vi "proc_append_error.vi"(8 "error in":errorcluster, 11 "code in":i32) -> (0 "error out":errorcluster, 3 "code out":i32)   [LabVIEW 2012]
doc: "Appends LV process error text to error signal."
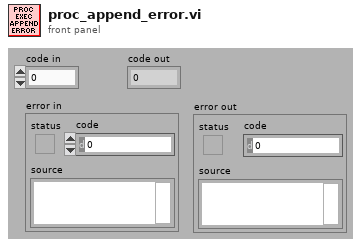
[diagram p1: front panel]
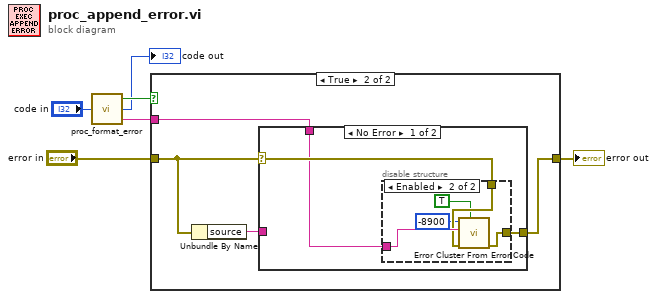
[diagram p0: block diagram]
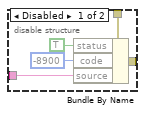
[diagram p3: hidden frame]
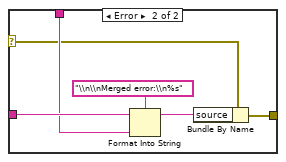
[diagram p4: hidden frame]
diagram:
  n1 = call "proc_format_error.vi"("code in"="code in") -> ("error"=w5:bool, "code out"=→"code out":i32, "error string"=w3:string)
  n2 = case shown="True" w5 {
    tunnel: "error in" -> [w7 w11]
    tunnel: w3 -> [_ w10]
    tunnel: [w7 w8] -> w2
    frame False {
    }
    frame True {
      n3 = Unbundle By Name(w11) -> ("source"=w9:string)
      n4 = case shown="No Error" w11 {
        selector: w11 -> [w14 w26]
        tunnel: w10 -> [w13 w28]
        tunnel: [w12 w25] -> w8
        tunnel: w9 -> [_ w30]
        frame No Error {
          n5 = disable-structure shown="Enabled" {
            disable-tunnel: w14 -> [w19 w23]
            disable-tunnel: w13 -> [w16 w24]
            disable-tunnel: [w15 w22] -> w12
            frame Disabled {
              n6 = Bundle By Name(cluster=w19, "status"=TRUE, "code"=-8900, "source"=w16) -> (w15:errorcluster)
            }
            frame Enabled {
              n7 = call <vilib>:"Error Cluster From Error Code.vi"("show call chain? (False)"=TRUE, "error in (no error)"=w23, "error message (\"\")"=w24, "error code (0)"=-8900) -> ("error out"=w22:errorcluster)  [unwired: 5 in]
            }
          }
        }
        frame Error {
          n8 = Format Into String(format string="\\n\\nMerged error:\\n%s", initial string=w30, w28) -> (resulting string=w27:string)  [unwired: 1 in, 1 out]
          n9 = Bundle By Name(cluster=w26, "source"=w27) -> (w25:errorcluster)
        }
      }
    }
  }
  "error out" <- w2
